vi "Actor Core.vi"(8 "error in":errorcluster, 11 "My Application":refnum<class "Manager.lvclass">) -> (0 "error out":errorcluster, 3 "Actor out":refnum<class "Actor.lvclass">)   [LabVIEW 2013, in "Manager.lvlib" / "Manager.lvclass"]
doc: "This is Actor Core.vi, the main message handling loop for Actors. An actor usually just sits in this loop and processes messages as they arrive. Any error returned by the message Do.vi call will stop the loop, with error code 43 as the canonical signal to stop with no error sent to caller. Descendants may override that in Handle Error.vi."
uses:
  Manager.lvclass
  PluginInterface/Actor Framework.lvlibp/Actor/Actor.lvclass
  Manager.lvclass/Manager.ctl
  Write System Ring Refnum.vi
  Write Actor Ring Refnum.vi
  Write Add Button Refnum.vi
  Write SubPnl Refnum.vi
  Write Remove Button Refnum.vi
  PluginInterface/Actor Framework.lvlibp/Message Enqueuer/Enqueue.vi
  Manager Messages/Add System Msg/Add System Msg.lvclass
  Manager Messages/Update SubPanel Msg/Update SubPanel Msg.lvclass
  Manager Messages/Remove System Msg/Remove System Msg.lvclass
  PluginInterface/Actor Framework.lvlibp/Stop Msg/Stop Msg.lvclass
panel:
  in  "stop signal":bool
  in  "Actor Ring":u16(ring) caption="View"
  in  "Add Button":bool
  in  "Remove Button":bool
  in  "System Ring":u16(ring)
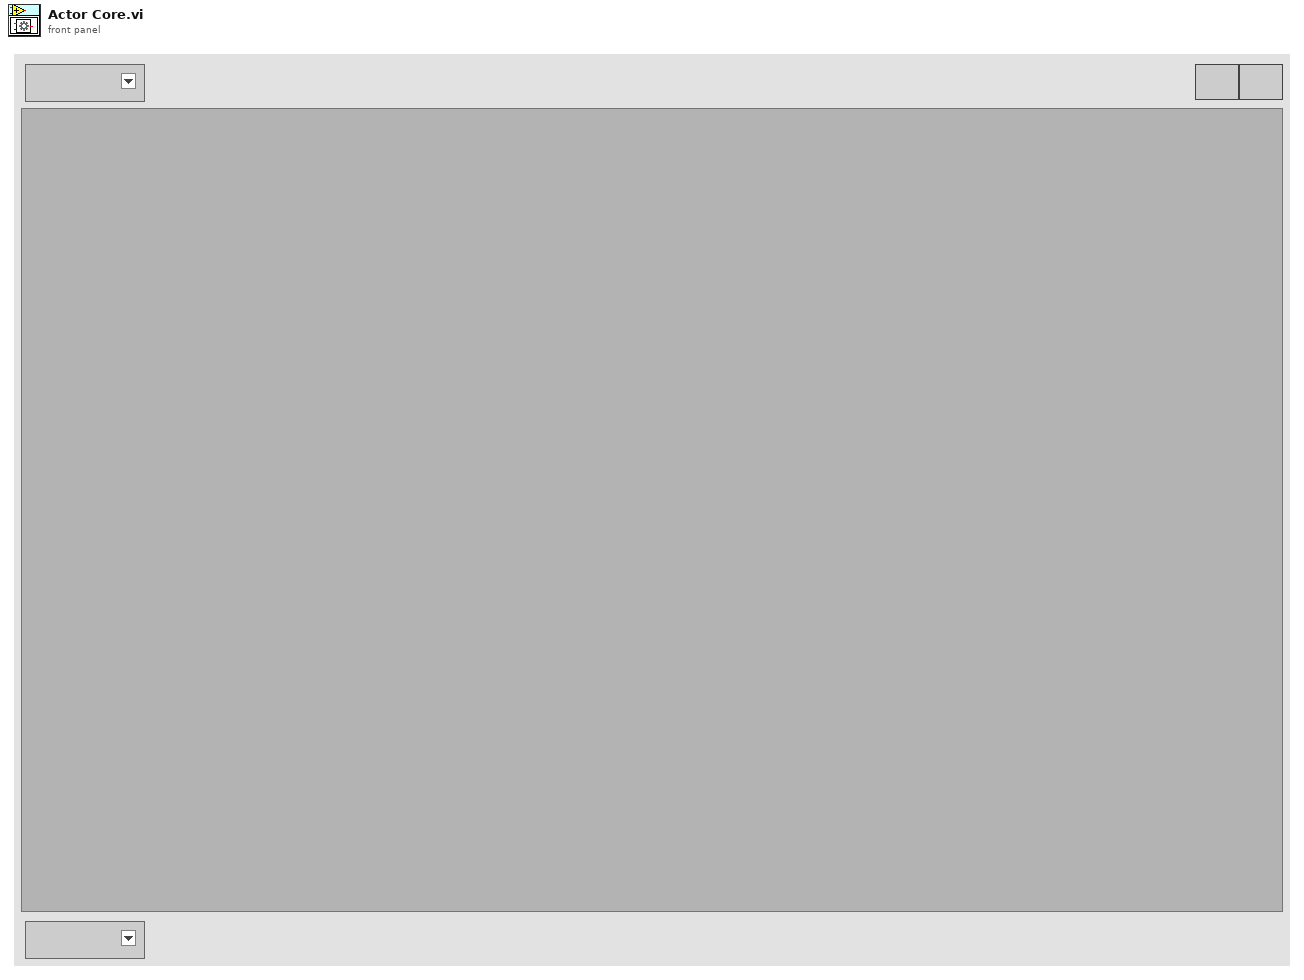
[diagram p1: front panel]
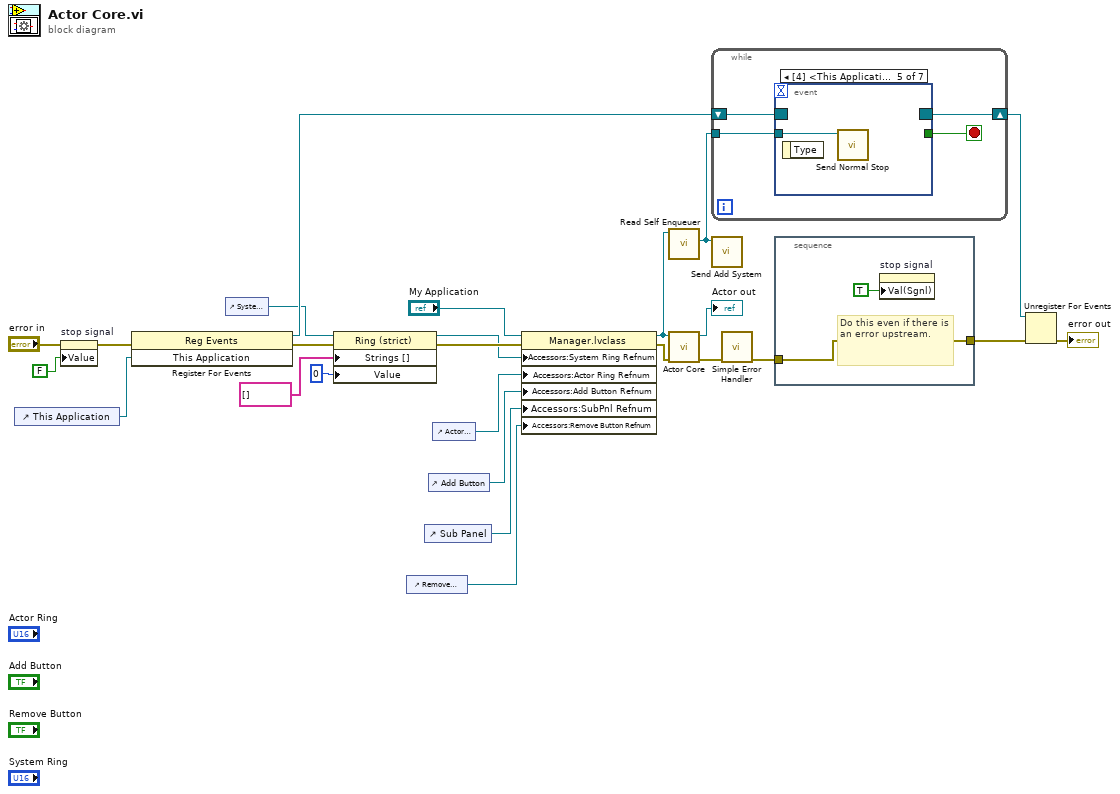
[diagram p0: block diagram]
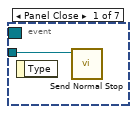
[diagram p2: hidden frame]
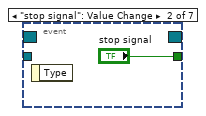
[diagram p3: hidden frame]
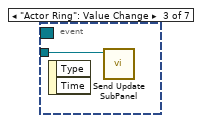
[diagram p4: hidden frame]
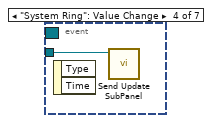
[diagram p5: hidden frame]
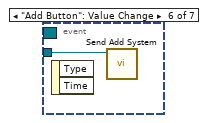
[diagram p6: hidden frame]
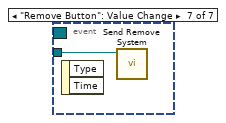
[diagram p7: hidden frame]
diagram:
  n1 = control-ref of="This Application"() -> (w16:refnum<vi>)
  n2 = property on="stop signal" class="Bool (strict)"(error in="error in", "Value"=FALSE ("stop")) -> (error out=w17:errorcluster)  [unwired: 1 in, 1 out]
  n3 = register-events(error in=w17, w16) -> (reference out=w21:refnum<event-registration>, error out=w7:errorcluster)  [unwired: 1 in]
  n4 = control-ref of="System Ring"() -> (w8:refnum<vi>)
  n5 = property class="Ring (strict)"(reference=w8, error in=w7, "Strings []"=string[] [], "Value"=0) -> (reference out=w3:refnum<vi>, error out=w4:errorcluster)
  n6 = control-ref of="Remove Button"() -> (w10:refnum<vi>)
  n7 = control-ref of="Sub Panel"() -> (w9:refnum<vi>)
  n8 = control-ref of="Add Button"() -> (w11:refnum<vi>)
  n9 = control-ref of="Actor Ring"() -> (w2:refnum<vi>)
  n10 = property class="Manager.lvclass"(reference="My Application", error in=w4, "Accessors:System Ring Refnum"=w3, "Accessors:Actor Ring Refnum"=w2, "Accessors:Add Button Refnum"=w11, "Accessors:SubPnl Refnum"=w9, "Accessors:Remove Button Refnum"=w10) -> (reference out=w12:refnum<class "Manager.lvclass">, error out=w14:errorcluster)
  n11 = call "Read Self Enqueuer.vi"("Actor"=w12) -> ("Self Enqueuer"=w1:refnum<class "Message Enqueuer.lvclass">)  [unwired: 10 in]
  n12 = call-parent "Actor Core.vi"("error in"=w14, "Actor in"=w12) -> ("error out"=w23:errorcluster, "Actor out"=→"Actor out":refnum<class "Actor.lvclass">)  [unwired: 8 in]
  n13 = while {
    tunnel: w1 -> [w29]
    shift-right: [w26] -> w20
    shift-left: w21 -> [w27]
    stop <- w28 stop-if-true
    n14 = event shown="[4] <This Application>: Application Instance Close" {
      selector: w27 -> [_ _ _ _ _ _ _]
      dyn-events: [_ _ _ _ _ _ _] -> w26
      timeout: _ -> [_ _ _ _ _ _ _]
      tunnel: w29 -> [w30 _ w32 w33 w34 w35 w36]
      tunnel: [_ "stop signal" _ _ _ _ _] -> w28
      event Panel Close {
        n15 = event-data() -> ()  [unwired: 1 in, 1 out]
        n16 = call "Send Normal Stop.vi"("Message Enqueuer"=w30) -> ()  [unwired: 10 in, 1 out]
      }
      event "stop signal": Value Change {
        n17 = event-data() -> ()  [unwired: 1 in, 1 out]
      }
      event "Actor Ring": Value Change {
        n18 = event-data() -> ()  [unwired: 1 in, 2 out]
        n19 = call "Send Update SubPanel.vi"("Message Enqueuer"=w32) -> ()  [unwired: 9 in, 2 out]
      }
      event "System Ring": Value Change {
        n20 = event-data() -> ()  [unwired: 1 in, 2 out]
        n21 = call "Send Update SubPanel.vi"("Message Enqueuer"=w33) -> ()  [unwired: 9 in, 2 out]
      }
      event Application Instance Close {
        n22 = event-data() -> ()  [unwired: 1 in, 1 out]
        n23 = call "Send Normal Stop.vi"("Message Enqueuer"=w34) -> ()  [unwired: 10 in, 1 out]
      }
      event "Add Button": Value Change {
        n24 = event-data() -> ()  [unwired: 1 in, 2 out]
        n25 = call "Send Add System.vi"("Message Enqueuer"=w35) -> ()  [unwired: 9 in, 2 out]
      }
      event "Remove Button": Value Change {
        n26 = event-data() -> ()  [unwired: 1 in, 2 out]
        n27 = call "Send Remove System.vi"("Message Enqueuer"=w36) -> ()  [unwired: 9 in, 2 out]
      }
    }
  }
  n28 = call "Send Add System.vi"("Message Enqueuer"=w1) -> ()  [unwired: 9 in, 2 out]
  n29 = call <vilib>:"Simple Error Handler.vi"("error in (no error)"=w23) -> ("error out"=w22:errorcluster)  [unwired: 4 in, 4 out]
  n30 = stacked-sequence {
    tunnel: [w37] -> w19
    tunnel: w22 -> [w37]
    frame #0 {
      # "Do this even if there is an error upstream."
      n31 = property on="stop signal" class="Bool (strict)"("Val(Sgnl)"=TRUE ("stop")) -> ()  [unwired: 2 in, 2 out]
    }
  }
  n32 = Unregister For Events(event registration refnum=w20, error in=w19) -> (error out=→"error out":errorcluster)
